vi "Interface_Dispatch_Get Parameter Control Refs.vi"(8 "error in (no error)":errorcluster, 11 "Interface_Dispatch in":refnum<class "Interface_Dispatch.lvclass">) -> (0 "error out":errorcluster, 1 "Dependencies Controls[]":refnum<vi>[](array[refnum]), 2 "Configuration Controls[]":refnum<vi>[](array[refnum]), 3 "Interface_Dispatch out":refnum<class "Interface_Dispatch.lvclass">, 4 "Output Controls[]":refnum<vi>[](array[refnum]))   [LabVIEW 2015, in "Interface_Dispatch.lvclass"]
uses:
  Interface_Dispatch.lvclass
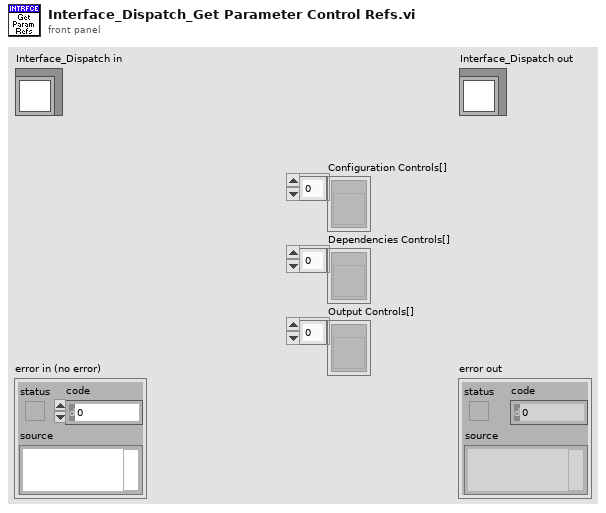
[diagram p1: front panel]
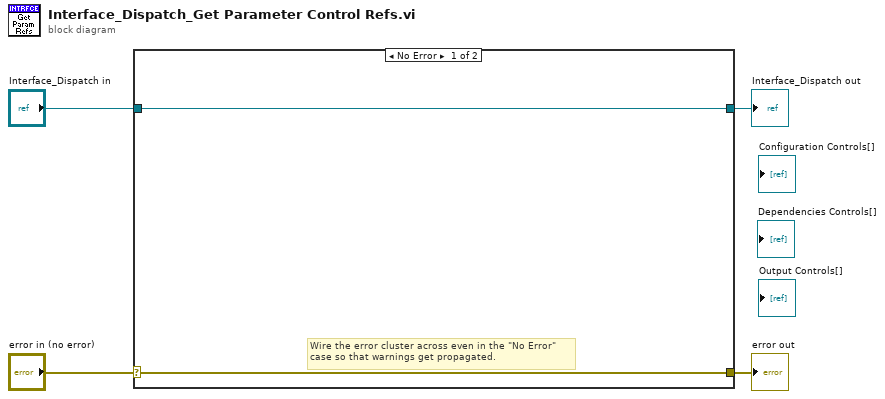
[diagram p0: block diagram]
diagram:
  n1 = case shown="No Error" "error in (no error)" {
    selector: "error in (no error)" -> [w5 w8]
    tunnel: [w5 w8] -> w3
    tunnel: [w6 w7] -> w1
    tunnel: "Interface_Dispatch in" -> [w6 w7]
    frame No Error {
      # "Wire the error cluster across even in the \"No Error\"\ncase so that warnings get propagated."
    }
    frame Error {
    }
  }
  "error out" <- w3
  "Interface_Dispatch out" <- w1
